vi "9264 16Ch Analog Output.vi"(2 "Packets":u64[](array[numeric])=[0, 0, 0, 0, 0, 0, 0, 0], 4 "9264 I/O":T1={"AO0"="NI 9264/AO0", "AO1"="NI 9264/AO1", "AO2"="NI 9264/AO2", "AO3"="NI 9264/AO3", "AO4"="NI 9264/AO4", "AO5"="NI 9264/AO5", "AO6"="NI 9264/AO6", "AO7"="NI 9264/AO7", "AO8"="NI 9264/AO8", "AO9"="NI 9264/AO9", "AO10"="NI 9264/AO10", "AO11"="NI 9264/AO11", "AO12"="NI 9264/AO12", "AO13"="NI 9264/AO13", "AO14"="NI 9264/AO14", "AO15"="NI 9264/AO15"}) -> ()   [LabVIEW 2010]
uses:
  <vilib>/eio/EIONode/EIONode.xnode
  <vilib>/rvi/eio/nirviEIOImplementation/nirviEIOImplementation.xnode
  <vilib>/rvi/eio/common/nirviEmuClasses.ctl
  <vilib>/rvi/eio/common/nirviEmuTemplateMethod_noerrors.vi
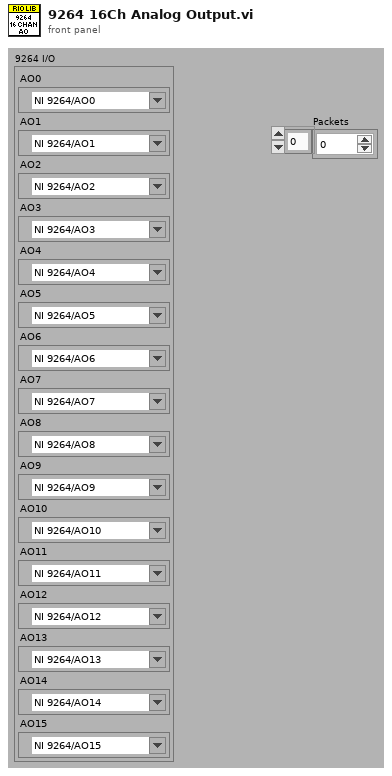
[diagram p1: front panel]
types:
  T1 = cluster{"AO0":refnum<k21>, "AO1":refnum<k21>, "AO2":refnum<k21>, "AO3":refnum<k21>, "AO4":refnum<k21>, "AO5":refnum<k21>, "AO6":refnum<k21>, "AO7":refnum<k21>, "AO8":refnum<k21>, "AO9":refnum<k21>, "AO10":refnum<k21>, "AO11":refnum<k21>, "AO12":refnum<k21>, "AO13":refnum<k21>, "AO14":refnum<k21>, "AO15":refnum<k21>}
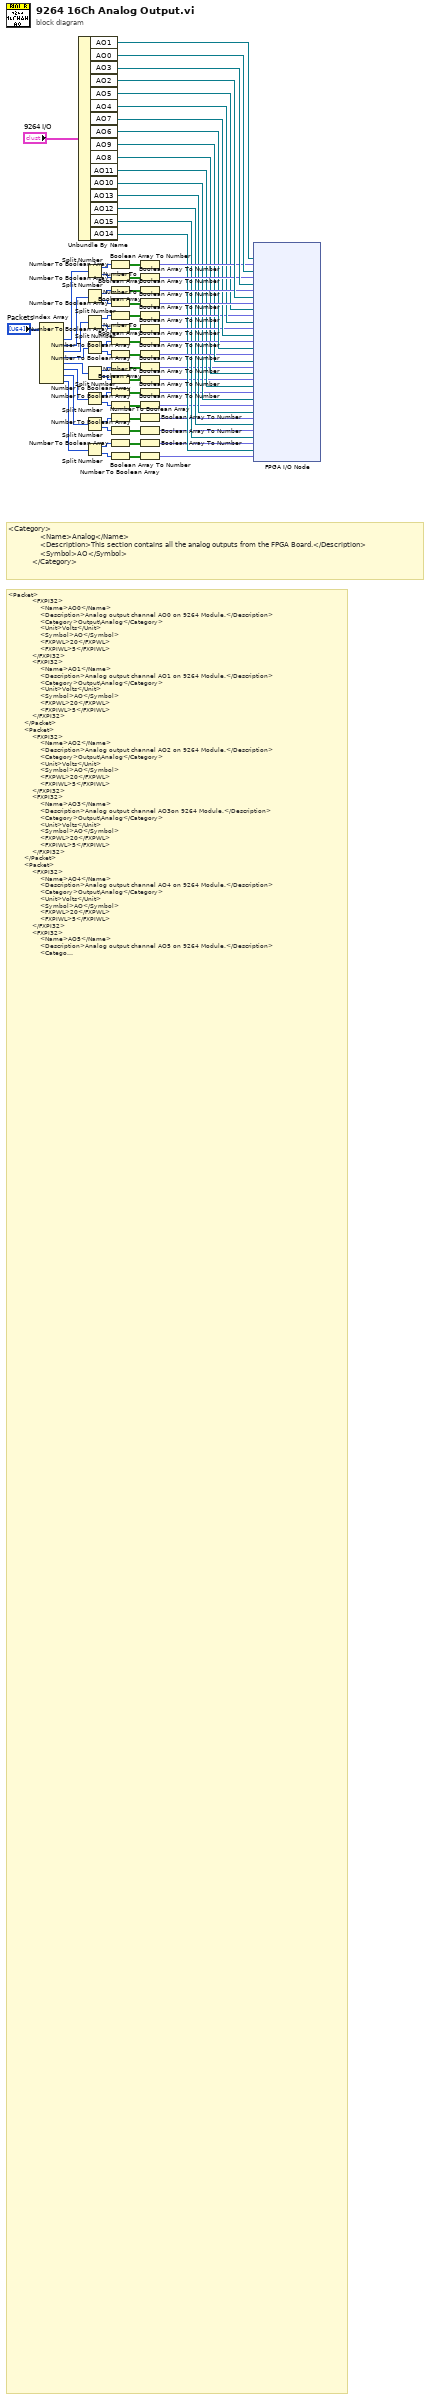
[diagram p0: block diagram]
diagram:
  # "<Category>\n                <Name>Analog</Name>\n                <Description>This section contains all the analog outputs from the FPGA Board.</Description>\n                <Symbol>AO</Symbol>\n            </Category>"
  # "<Packet>\n            <FXPI32>\n                <Name>AO0</Name>\n                <Description>Analog output channel AO0 on 9264 Module.</Description>\n                <Category>Output\\Analog</Category>\n                <Unit>Volts</Unit>\n                <Symbol>AO</Symbol>\n                <FXPWL>20</FXPWL>\n                <FXPIWL>5</FXPIWL>\n            </FXPI32>\n            <FXPI32>\n                <Name>AO1</Name>\n                <Description>Analog output channel AO1 on 9264 Module.</Description>\n                <Category>Output\\Analog</Category>\n                <Unit>Volts</Unit>\n                <Symbol>AO</Symbol>\n                <FXPWL>20</FXPWL>\n                <FXPIWL>5</FXPIWL>\n            </FXPI32>\n        </Packet>\n        <Packet>\n            <FXPI32>\n                <Name>AO2</Name>\n                <Description>Analog output channel AO2 on 9264 Module.</Description>\n                <Category>Output\\Analog</Category>\n                <Unit>Volts</Unit>\n                <Symbol>AO</Symbol>\n                <FXPWL>20</FXPWL>\n                <FXPIWL>5</FXPIWL>\n            </FXPI32>\n            <FXPI32>\n                <Name>AO3</Name>\n                <Description>Analog output channel AO3on 9264 Module.</Description>\n                <Category>Output\\Analog</Category>\n                <Unit>Volts</Unit>\n                <Symbol>AO</Symbol>\n                <FXPWL>20</FXPWL>\n                <FXPIWL>5</FXPIWL>\n            </FXPI32>\n        </Packet>\n        <Packet>\n            <FXPI32>\n                <Name>AO4</Name>\n                <Description>Analog output channel AO4 on 9264 Module.</Description>\n                <Category>Output\\Analog</Category>\n                <Unit>Volts</Unit>\n                <Symbol>AO</Symbol>\n                <FXPWL>20</FXPWL>\n                <FXPIWL>5</FXPIWL>\n            </FXPI32>\n            <FXPI32>\n                <Name>AO5</Name>\n                <Description>Analog output channel AO5 on 9264 Module.</Description>\n                <Category>Output\\Analog</Category>\n                <Unit>Volts</Unit>\n                <Symbol>AO</Symbol>\n                <FXPWL>20</FXPWL>\n                <FXPIWL>5</FXPIWL>\n            </FXPI32>\n        </Packet>\n        <Packet>\n            <FXPI32>\n                <Name>AO6</Name>\n                <Description>Analog output channel AO6 on 9264 Module.</Description>\n                <Category>Output\\Analog</Category>\n                <Unit>Volts</Unit>\n                <Symbol>AO</Symbol>\n                <FXPWL>20</FXPWL>\n                <FXPIWL>5</FXPIWL>\n            </FXPI32>\n            <FXPI32>\n                <Name>AO7</Name>\n                <Description>Analog output channel AO7on 9264 Module.</Description>\n                <Category>Output\\Analog</Category>\n                <Unit>Volts</Unit>\n                <Symbol>AO</Symbol>\n                <FXPWL>20</FXPWL>\n                <FXPIWL>5</FXPIWL>\n            </FXPI32>\n        </Packet>\n        <Packet>\n            <FXPI32>\n                <Name>AO8</Name>\n                <Description>Analog output channel AO8 on 9264 Module.</Description>\n                <Category>Output\\Analog</Category>\n                <Unit>Volts</Unit>\n                <Symbol>AO</Symbol>\n                <FXPWL>20</FXPWL>\n                <FXPIWL>5</FXPIWL>\n            </FXPI32>\n            <FXPI32>\n                <Name>AO9</Name>\n                <Description>Analog output channel AO9 on 9264 Module.</Description>\n                <Category>Output\\Analog</Category>\n                <Unit>Volts</Unit>\n                <Symbol>AO</Symbol>\n                <FXPWL>20</FXPWL>\n                <FXPIWL>5</FXPIWL>\n            </FXPI32>\n        </Packet>\n        <Packet>\n            <FXPI32>\n                <Name>AO10</Name>\n                <Description>Analog output channel AO10 on 9264 Module.</Description>\n                <Category>Output\\Analog</Category>\n                <Unit>Volts</Unit>\n                <Symbol>AO</Symbol>\n                <FXPWL>20</FXPWL>\n                <FXPIWL>5</FXPIWL>\n            </FXPI32>\n            <FXPI32>\n                <Name>AO11</Name>\n                <Description>Analog output channel AO11 on 9264 Module.</Description>\n                <Category>Output\\Analog</Category>\n                <Unit>Volts</Unit>\n                <Symbol>AO</Symbol>\n                <FXPWL>20</FXPWL>\n                <FXPIWL>5</FXPIWL>\n            </FXPI32>\n        </Packet>\n        <Packet>\n            <FXPI32>\n                <Name>AO12</Name>\n                <Description>Analog output channel AO12 on 9264 Module.</Description>\n                <Category>Output\\Analog</Category>\n                <Unit>Volts</Unit>\n                <Symbol>AO</Symbol>\n                <FXPWL>20</FXPWL>\n                <FXPIWL>5</FXPIWL>\n            </FXPI32>\n            <FXPI32>\n                <Name>AO13</Name>\n                <Description>Analog output channel AO13 on 9264 Module.</Description>\n                <Category>Output\\Analog</Category>\n                <Unit>Volts</Unit>\n                <Symbol>AO</Symbol>\n                <FXPWL>20</FXPWL>\n                <FXPIWL>5</FXPIWL>\n            </FXPI32>\n        </Packet>\n        <Packet>\n            <FXPI32>\n                <Name>AO14</Name>\n                <Description>Analog output channel AO14 on 9264 Module.</Description>\n                <Category>Output\\Analog</Category>\n                <Unit>Volts</Unit>\n                <Symbol>AO</Symbol>\n                <FXPWL>20</FXPWL>\n                <FXPIWL>5</FXPIWL>\n            </FXPI32>\n            <FXPI32>\n                <Name>AO15</Name>\n                <Description>Analog output channel AO15on 9264 Module.</Description>\n                <Category>Output\\Analog</Category>\n                <Unit>Volts</Unit>\n                <Symbol>AO</Symbol>\n                <FXPWL>20</FXPWL>\n                <FXPIWL>5</FXPIWL>\n            </FXPI32>\n        </Packet>"
  n1 = Index Array(array="Packets") -> (element #1=w56:u64, element #2=w57:u64, element #3=w39:u64, element #4=w38:u64, element #5=w4:u64, element #6=w1:u64, element #7=w2:u64, element #8=w3:u64)  [unwired: 8 in]
  n2 = Unbundle By Name("9264 I/O") -> ("AO1"=w73:refnum<k21>, "AO0"=w74:refnum<k21>, "AO3"=w72:refnum<k21>, "AO2"=w71:refnum<k21>, "AO5"=w46:refnum<k21>, "AO4"=w45:refnum<k21>, "AO7"=w44:refnum<k21>, "AO6"=w43:refnum<k21>, "AO9"=w37:refnum<k21>, "AO8"=w35:refnum<k21>, "AO11"=w34:refnum<k21>, "AO10"=w33:refnum<k21>, "AO13"=w32:refnum<k21>, "AO12"=w31:refnum<k21>, "AO15"=w30:refnum<k21>, "AO14"=w29:refnum<k21>)
  n3 = Split Number(x=w56) -> (hi(x)=w58:u32, lo(x)=w59:u32)
  n4 = Split Number(x=w57) -> (hi(x)=w60:u32, lo(x)=w61:u32)
  n5 = Split Number(x=w39) -> (hi(x)=w54:u32, lo(x)=w53:u32)
  n6 = Split Number(x=w38) -> (hi(x)=w52:u32, lo(x)=w51:u32)
  n7 = Split Number(x=w4) -> (hi(x)=w20:u32, lo(x)=w19:u32)
  n8 = Split Number(x=w1) -> (hi(x)=w18:u32, lo(x)=w17:u32)
  n9 = Split Number(x=w2) -> (hi(x)=w21:u32, lo(x)=w22:u32)
  n10 = Split Number(x=w3) -> (hi(x)=w23:u32, lo(x)=w24:u32)
  n11 = Number To Boolean Array(number=w58) -> (Boolean array=w63:bool[])
  n12 = Number To Boolean Array(number=w59) -> (Boolean array=w65:bool[])
  n13 = Number To Boolean Array(number=w60) -> (Boolean array=w66:bool[])
  n14 = Number To Boolean Array(number=w61) -> (Boolean array=w68:bool[])
  n15 = Number To Boolean Array(number=w54) -> (Boolean array=w50:bool[])
  n16 = Number To Boolean Array(number=w53) -> (Boolean array=w49:bool[])
  n17 = Number To Boolean Array(number=w52) -> (Boolean array=w48:bool[])
  n18 = Number To Boolean Array(number=w51) -> (Boolean array=w47:bool[])
  n19 = Number To Boolean Array(number=w20) -> (Boolean array=w16:bool[])
  n20 = Number To Boolean Array(number=w19) -> (Boolean array=w15:bool[])
  n21 = Number To Boolean Array(number=w18) -> (Boolean array=w14:bool[])
  n22 = Number To Boolean Array(number=w17) -> (Boolean array=w13:bool[])
  n23 = Number To Boolean Array(number=w21) -> (Boolean array=w25:bool[])
  n24 = Number To Boolean Array(number=w22) -> (Boolean array=w26:bool[])
  n25 = Number To Boolean Array(number=w23) -> (Boolean array=w27:bool[])
  n26 = Number To Boolean Array(number=w24) -> (Boolean array=w28:bool[])
  n27 = Boolean Array To Number(Boolean array=w63) -> (number=w62:fxp<+/-,20,5>)
  n28 = Boolean Array To Number(Boolean array=w65) -> (number=w64:fxp<+/-,20,5>)
  n29 = Boolean Array To Number(Boolean array=w66) -> (number=w67:fxp<+/-,20,5>)
  n30 = Boolean Array To Number(Boolean array=w68) -> (number=w69:fxp<+/-,20,5>)
  n31 = Boolean Array To Number(Boolean array=w50) -> (number=w40:fxp<+/-,20,5>)
  n32 = Boolean Array To Number(Boolean array=w49) -> (number=w41:fxp<+/-,20,5>)
  n33 = Boolean Array To Number(Boolean array=w48) -> (number=w42:fxp<+/-,20,5>)
  n34 = Boolean Array To Number(Boolean array=w47) -> (number=w36:fxp<+/-,20,5>)
  n35 = Boolean Array To Number(Boolean array=w16) -> (number=w5:fxp<+/-,20,5>)
  n36 = Boolean Array To Number(Boolean array=w15) -> (number=w6:fxp<+/-,20,5>)
  n37 = Boolean Array To Number(Boolean array=w14) -> (number=w7:fxp<+/-,20,5>)
  n38 = Boolean Array To Number(Boolean array=w13) -> (number=w8:fxp<+/-,20,5>)
  n39 = Boolean Array To Number(Boolean array=w25) -> (number=w9:fxp<+/-,20,5>)
  n40 = Boolean Array To Number(Boolean array=w26) -> (number=w10:fxp<+/-,20,5>)
  n41 = Boolean Array To Number(Boolean array=w27) -> (number=w11:fxp<+/-,20,5>)
  n42 = Boolean Array To Number(Boolean array=w28) -> (number=w12:fxp<+/-,20,5>)
  n43 = xnode "FPGA I/O Node"("I/O Item"=w62, "I/O Item"=w64, "I/O Item"=w67, "I/O Item"=w69, "I/O Item"=w40, "I/O Item"=w41, "I/O Item"=w42, "I/O Item"=w36, "I/O Item"=w5, "I/O Item"=w6, "I/O Item"=w7, "I/O Item"=w8, "I/O Item"=w9, "I/O Item"=w10, "I/O Item"=w11, "I/O Item"=w12, "FPGA I/O In"=w73, "FPGA I/O In"=w74, "FPGA I/O In"=w72, "FPGA I/O In"=w71, "FPGA I/O In"=w46, "FPGA I/O In"=w45, "FPGA I/O In"=w44, "FPGA I/O In"=w43, "FPGA I/O In"=w37, "FPGA I/O In"=w35, "FPGA I/O In"=w34, "FPGA I/O In"=w33, "FPGA I/O In"=w32, "FPGA I/O In"=w31, "FPGA I/O In"=w30, "FPGA I/O In"=w29) -> ()  [unwired: 16 out]
